vi "Robot Information Global.vi"() -> ()   [LabVIEW 2018]
panel:
  out "Testglobal":bool
  in  "Robot Size":cluster{"Robot Width":dbl, "Robot Length":dbl}={"Robot Width"=21.5, "Robot Length"=25.5}
  in  "Cargo State":enum16{""}(ring)
  in  "Hatch Pannel State":enum16{""}(ring)
  in  "Lift State":enum16{""}(ring)
  in  "HAB Climber State":enum16{""}(ring)
  out "Practice Robot":bool
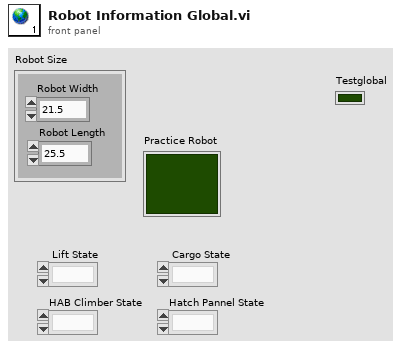
[diagram p1: front panel]
diagram:
